vi "getAllParagraphs.vi"(8 "error in (no error)":errorcluster, 11 "xwpfWriter in":refnum<class "xwpfWriter.lvclass">=refnum) -> (0 "error out":errorcluster, 2 "All Paragraphs":string[](array[string]), 3 "xwpfWriter out":refnum<class "xwpfWriter.lvclass">)   [LabVIEW 2017, in "LabVIEW NPOI.lvlib" / "xwpfWriter.lvclass"]
uses:
  xwpfWriter.lvclass
  xwpfWriter.lvclass/xwpfWriter.ctl
  C:/Users/Neo/Desktop/Dev_Tools_BR/LabVIEW_NPOI/src/lib/NPOI 2.1.1/NPOI.OOXML.dll
  lib/NPOI 2.1.1/NPOI.OOXML.dll
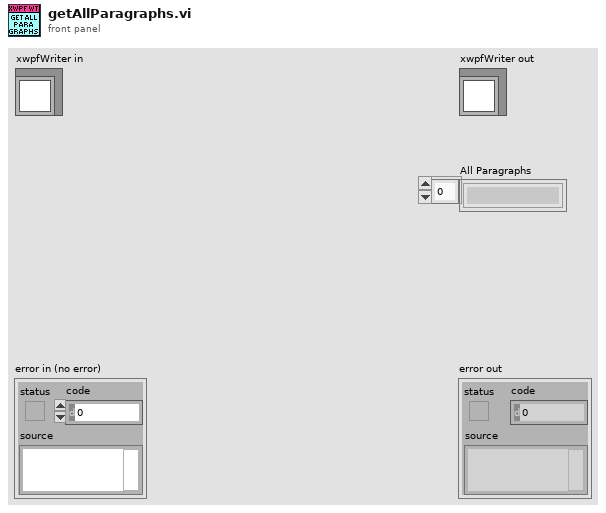
[diagram p1: front panel]
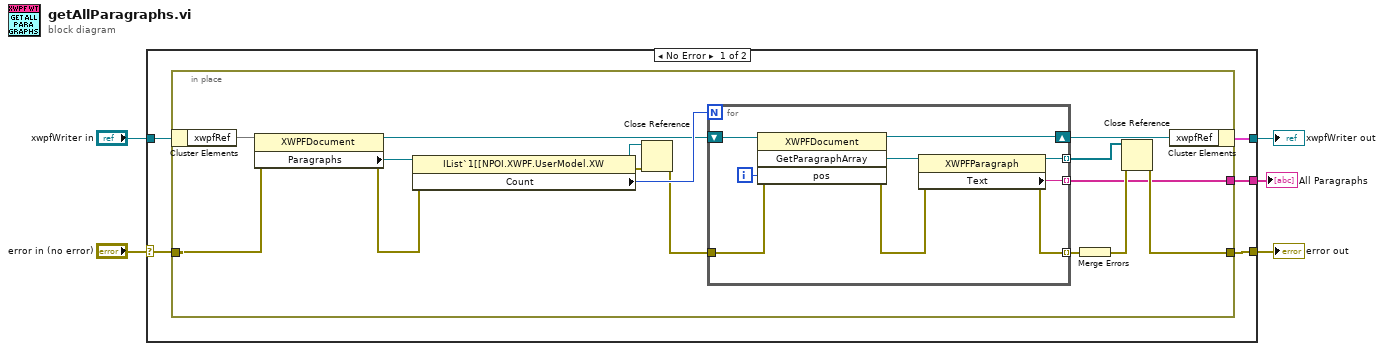
[diagram p0: block diagram]
diagram:
  n1 = case shown="No Error" "error in (no error)" {
    selector: "error in (no error)" -> [w9 w36]
    tunnel: [w7 w36] -> w4
    tunnel: [w8 w35] -> w2
    tunnel: "xwpfWriter in" -> [w10 w35]
    tunnel: [w6 _] -> w1
    frame No Error {
      n2 = in-place {
        in-place-border: w9 -> [w22]
        in-place-border: [w13] -> w7
        in-place-border: [w11] -> w6
        n3 = in-place-cluster #1(w10) -> ("xwpfRef"=w25)
        n4 = property class="XWPFDocument"(reference=w25, error in=w22) -> (reference out=w21:refnum<k24>, error out=w18:errorcluster, "Paragraphs"=w24:refnum<k24>)
        n5 = property class="IList`1[[NPOI.XWPF.UserModel.XW"(reference=w24, error in=w18) -> (reference out=w17:refnum<k24>, error out=w16:errorcluster, "Count"=w23:i32)
        n6 = Close Reference(reference=w17, error in (no error)=w16) -> (error out=w15:errorcluster)
        n7 = for {
          N: w23 -> [_]
          tunnel: [w29] -> w11 mode=indexing
          tunnel: [w26] -> w14 mode=indexing
          shift-right: [w33] -> w20
          shift-left: w21 -> [w31]
          tunnel: w15 -> [w32]
          tunnel: [w27] -> w19 mode=indexing
          i -> [w34]
          n8 = invoke class="XWPFDocument" method="GetParagraphArray"(reference=w31, error in=w32, "pos"=w34) -> (reference out=w33:refnum<k24>, error out=w28:errorcluster, "GetParagraphArray"=w30:refnum<k24>)  [unwired: 1 in, 1 out]
          n9 = property class="XWPFParagraph"(reference=w30, error in=w28) -> (reference out=w26:refnum<k24>, error out=w27:errorcluster, "Text"=w29:string)
        }
        n10 = Merge Errors(w19) -> (w12:errorcluster)
        n11 = Close Reference(reference=w14, error in (no error)=w12) -> (error out=w13:errorcluster)
        n12 = in-place-cluster #1("xwpfRef"=w20) -> (w8:cluster{})
      }
    }
    frame Error {
    }
  }
  "error out" <- w4
  "xwpfWriter out" <- w2
  "All Paragraphs" <- w1
